vi "Update Worker Status MHLC.vi"(8 "error in (no error)":errorcluster, 10 "Data in":variant, 11 "AppMgr in":refnum<class "Application Manager.lvclass">) -> (0 "error out":errorcluster, 3 "AppMgr out":refnum<class "Application Manager.lvclass">)   [LabVIEW 2017, in "Application Manager.lvclass"]
doc: "Update the status of the Worker in the tree"
uses:
  Application Manager.lvclass
  C:/Program Files (x86)/National Instruments/LabVIEW 2017/vi.lib/addons/_Workers/Library/Classes/Worker/Worker.lvclass
  <vilib>/addons/_Workers/Library/Classes/Worker/Worker Status Data.ctl
  <vilib>/addons/_Workers/Library/Classes/Worker/Worker Status.ctl
  <vilib>/addons/_Workers/Library/Classes/Worker/Worker.lvclass/Worker.ctl
  <vilib>/addons/_Workers/Library/Classes/Message/Message.lvclass/Message.ctl
  Application Manager.lvclass/Application Manager.ctl
  <vilib>/addons/_Workers/Library/Classes/Worker/Read Message.vi
  <vilib>/addons/_Workers/Library/Classes/Message/Read Sender WID.vi
  Common VIs/DC Name to DC_UID.vi
  <vilib>/Utility/error.llb/Error Cluster From Error Code.vi
  <vilib>/ErrorRing/Error Ring.xnode
  <vilib>/addons/_Workers/Library/Classes/Worker/Worker.lvclass
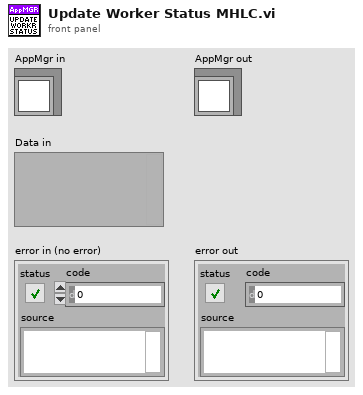
[diagram p1: front panel]
types:
  T1 = typedef "Workers.lvlib/Worker.lvclass/Worker Status Data.ctl" = cluster{"WID":string, "Worker Status":T2, "Custom User Status":string}
  T2 = typedef "Workers.lvlib/Worker.lvclass/Worker Status.ctl" = enum16{"Queue created", "Preinitialized", "Initialize called", "Initialized", "Start Exiting called", "Exited", "Stopped (Critical Error)"}
  T3 = typedef "DC_UID.ctl" = string
  T4 = typedef "Application Manager.lvclass/Debug Client Data.ctl" = cluster{"DC_UID":T3, "IP Address":string, "Worker Data":T5[], "Connected":bool}
  T5 = typedef "Application Manager.lvclass/Worker Data.ctl" = cluster{"ID":string, "VI Ref":refnum<vi>, "VI Path":path, "CloneID":string, "Type":T6, "Worker Status":string}
  T6 = typedef "Workers.lvlib/Worker.lvclass/Worker Type.ctl" = enum16{"SL", "DL"}
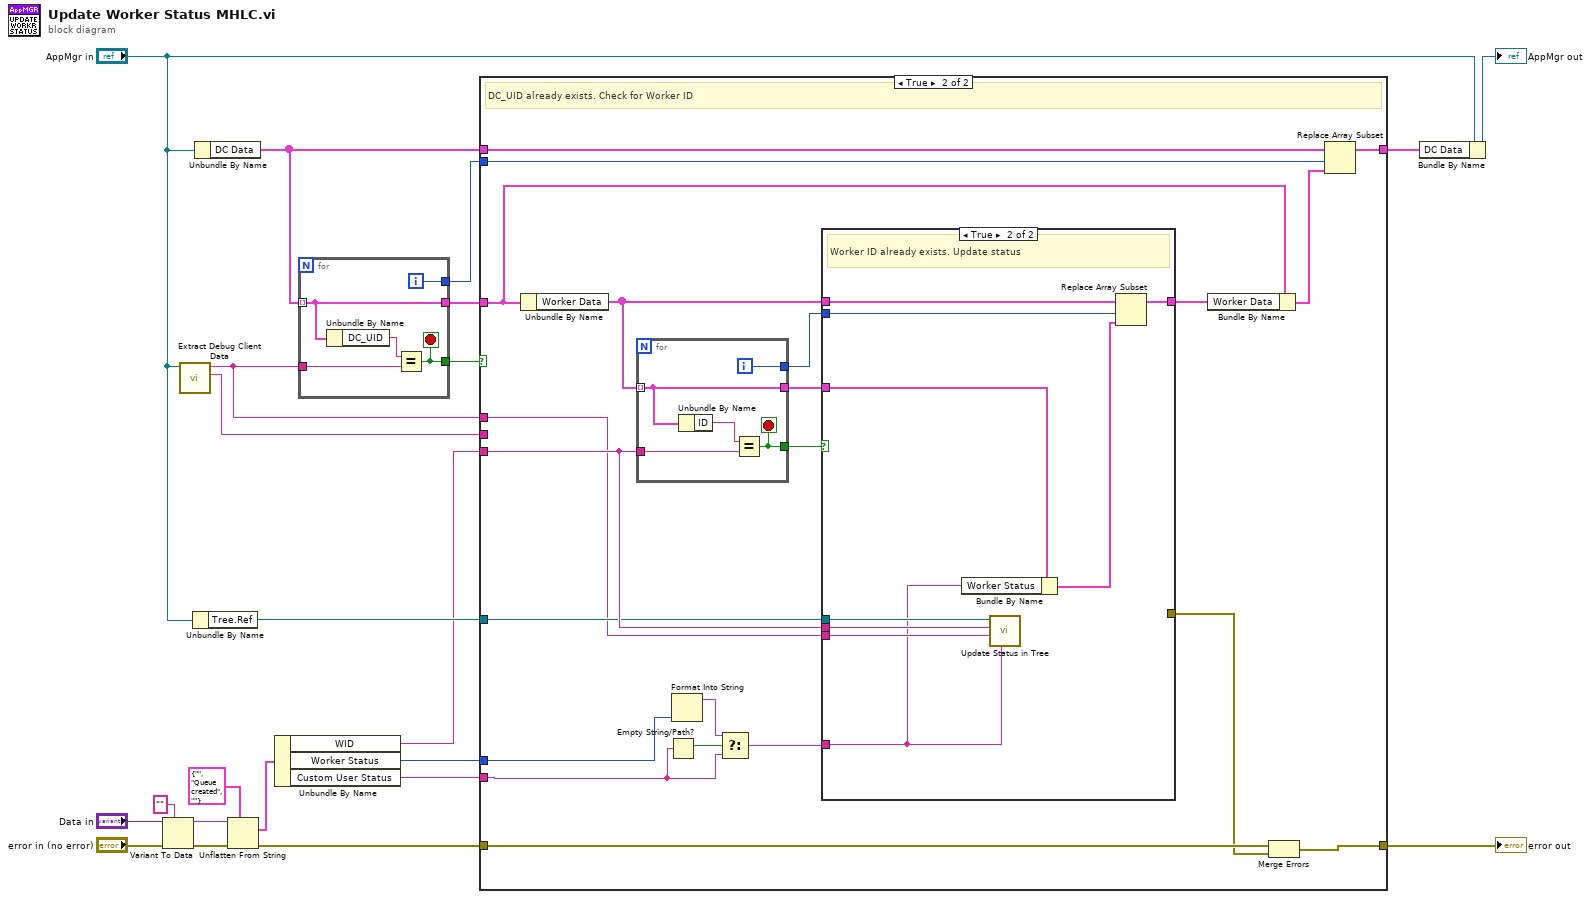
[diagram p0: block diagram]
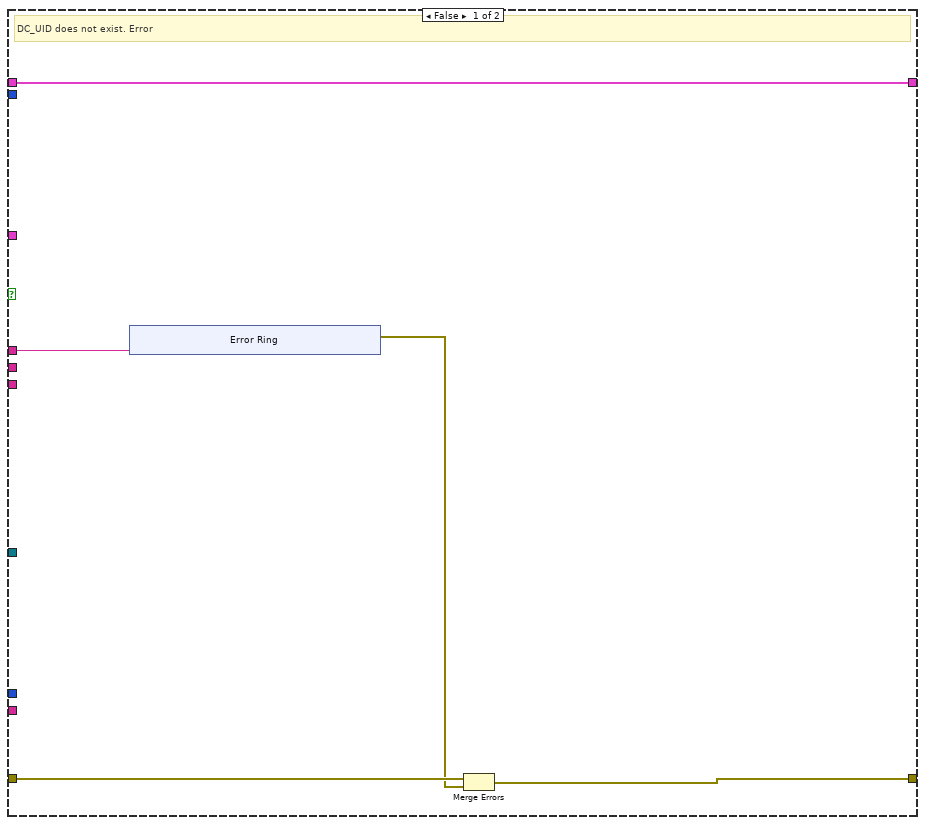
[diagram p2: hidden frame]
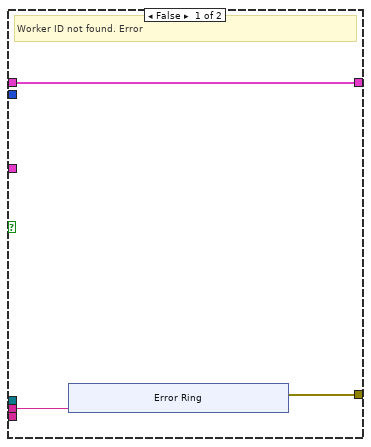
[diagram p3: hidden frame]
diagram:
  n1 = Variant To Data(error in="error in (no error)", type="", Variant="Data in") -> (data=w20:string, error out=w21:errorcluster)
  n2 = call "Extract Debug Client Data.vi"("AppMgr in"="AppMgr in") -> ("IP Address"=w17:string, "DC_UID"=w18:T3)  [unwired: 9 in]
  n3 = Unbundle By Name("AppMgr in") -> ("Tree.Ref"=w16:refnum<vi>)
  n4 = Unbundle By Name("AppMgr in") -> ("DC Data"=w19:T4[])
  n5 = Unflatten From String(type=T1 {"WID"="", "Worker Status"=enum."Queue created", "Custom User Status"=""} ("Worker Status Data"), binary string=w20, error in (no error)=w21) -> (value=w11:T1, error out=w9:errorcluster)  [unwired: 2 in, 1 out]
  n6 = Unbundle By Name(w11) -> ("WID"=w10:string, "Worker Status"=w8:T2, "Custom User Status"=w7:string)
  n7 = for {
    tunnel: w19 -> [w23] mode=indexing
    tunnel: w18 -> [w26]
    tunnel: [w25] -> w12
    tunnel: [w24] -> w15
    tunnel: [w23] -> w13
    i -> [w24]
    stop <- w25 stop-if-true
    n8 = Unbundle By Name(w23) -> ("DC_UID"=w27:T3)
    n9 = Equal?(x=w27, y=w26) -> (x = y?=w25:bool)
  }
  n10 = case shown="True" w12 {
    tunnel: w19 -> [w32 w60]
    tunnel: w18 -> [w28 w48]
    tunnel: w10 -> [_ w51]
    tunnel: w17 -> [_ _]
    tunnel: w16 -> [_ w49]
    tunnel: w15 -> [_ w58]
    tunnel: [w32 w59] -> w14
    tunnel: w13 -> [_ w56]
    tunnel: [w30 w46] -> w2
    tunnel: w9 -> [w31 w47]
    tunnel: w8 -> [_ w42]
    tunnel: w7 -> [_ w41]
    frame False {
      # "DC_UID does not exist. Error"
      n11 = xnode "Error Ring"("parameter 0"=w28) -> ("error out"=w29:errorcluster)
      n12 = Merge Errors(w31, w29) -> (w30:errorcluster)
    }
    frame True {
      # "DC_UID already exists. Check for Worker ID"
      n13 = Unbundle By Name(w56) -> ("Worker Data"=w54:T5[])
      n14 = for {
        tunnel: w54 -> [w80] mode=indexing
        tunnel: w51 -> [w83]
        tunnel: [w82] -> w57
        tunnel: [w81] -> w52
        tunnel: [w80] -> w50
        i -> [w81]
        stop <- w82 stop-if-true
        n15 = Unbundle By Name(w80) -> ("ID"=w84:string)
        n16 = Equal?(x=w84, y=w83) -> (x = y?=w82:bool)
      }
      n17 = Empty String/Path?(string/path=w41) -> (empty?=w44:bool)
      n18 = Format Into String(w42) -> (resulting string=w43:string)  [unwired: 3 in, 1 out]
      n19 = Select(t=w43, s=w44, f=w41) -> (s? t:f=w40:string)
      n20 = case shown="True" w57 {
        tunnel: w54 -> [w63 w79]
        tunnel: [w63 w78] -> w53
        tunnel: w52 -> [_ w77]
        tunnel: w51 -> [w62 w73]
        tunnel: w50 -> [_ w76]
        tunnel: w49 -> [_ w74]
        tunnel: w48 -> [_ w72]
        tunnel: [w61 _] -> w45
        tunnel: w40 -> [_ w71]
        frame False {
          # "Worker ID not found. Error"
          n21 = xnode "Error Ring"("parameter 0"=w62) -> ("error out"=w61:errorcluster)
        }
        frame True {
          # "Worker ID already exists. Update status"
          n22 = Bundle By Name(cluster=w76, "Worker Status"=w71) -> (w75:T5)
          n23 = call "Update Status in Tree.vi"("Worker Status"=w71, "DC_UID"=w72, "WID"=w73, "Tree Ref"=w74) -> ()  [unwired: 7 in, 1 out]
          n24 = Replace Array Subset(array=w79, new element=w75, index=w77) -> (w78:T5[])
        }
      }
      n25 = Bundle By Name(cluster=w56, "Worker Data"=w53) -> (w55:T4)
      n26 = Merge Errors(w47, w45) -> (w46:errorcluster)
      n27 = Replace Array Subset(array=w60, new element=w55, index=w58) -> (w59:T4[])
    }
  }
  "error out" <- w2
  n28 = Bundle By Name(cluster="AppMgr in", "DC Data"=w14) -> (→"AppMgr out":refnum<class "Application Manager.lvclass">)
